vi "UA_Add node.vi"(8 "error in (no error)":errorcluster caption="错误输入（无错误）", 9 "XML Folder":T2[](array[typedef]), 11 "OPC UA server refnum in":refnum<k21>) -> (0 "error out":errorcluster caption="错误输出", 3 "OPC UA server refnum out":refnum<k21>)   [LabVIEW 2013, in "OPCUA XML.lvlib"]
uses:
  OPCUA XML.lvlib
  UA_XML Data.ctl
  UA_RowType.ctl
  UA_Node.ctl
  UA_OP Action.ctl
  <vilib>/OPCUA/NI OPC UA Server.lvlib
panel:
  out "node out":T1
  out "Data":string
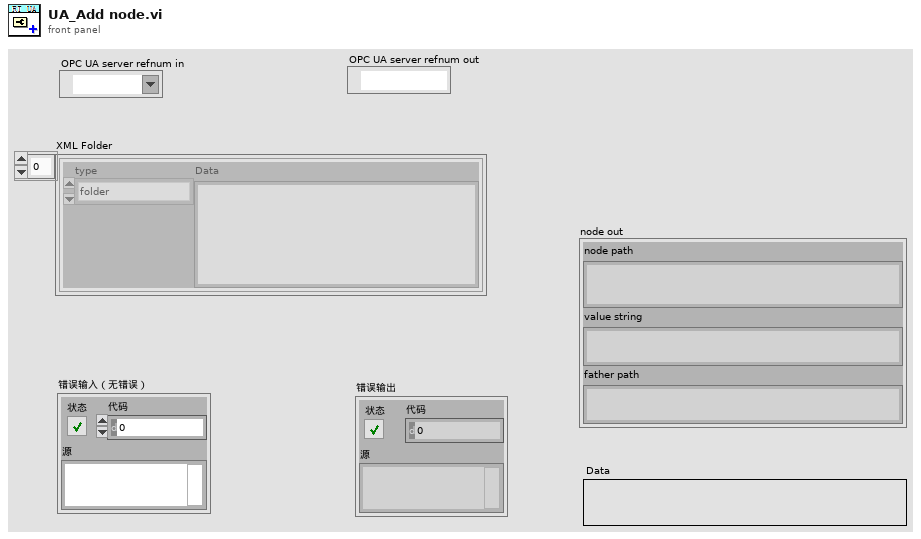
[diagram p1: front panel]
types:
  T1 = typedef "OPCUA XML.lvlib/UA_Node.ctl" = cluster{"node path":string, "value string":string, "father path":string}
  T2 = typedef "OPCUA XML.lvlib/UA_XML Data.ctl" = cluster{"type":T3, "Data":string}
  T3 = typedef "OPCUA XML.lvlib/UA_RowType.ctl" = enum16{"none", "folder", "item", "property", "folder end", "item end"}
  T4 = typedef "OPCUA XML.lvlib/UA_OP Action.ctl" = enum16{"Initial", "Add node", "Get node", "Get length", "View node"}
  T5 = cluster{"name":string, "data type":u16, "access level":u16, "description":string}
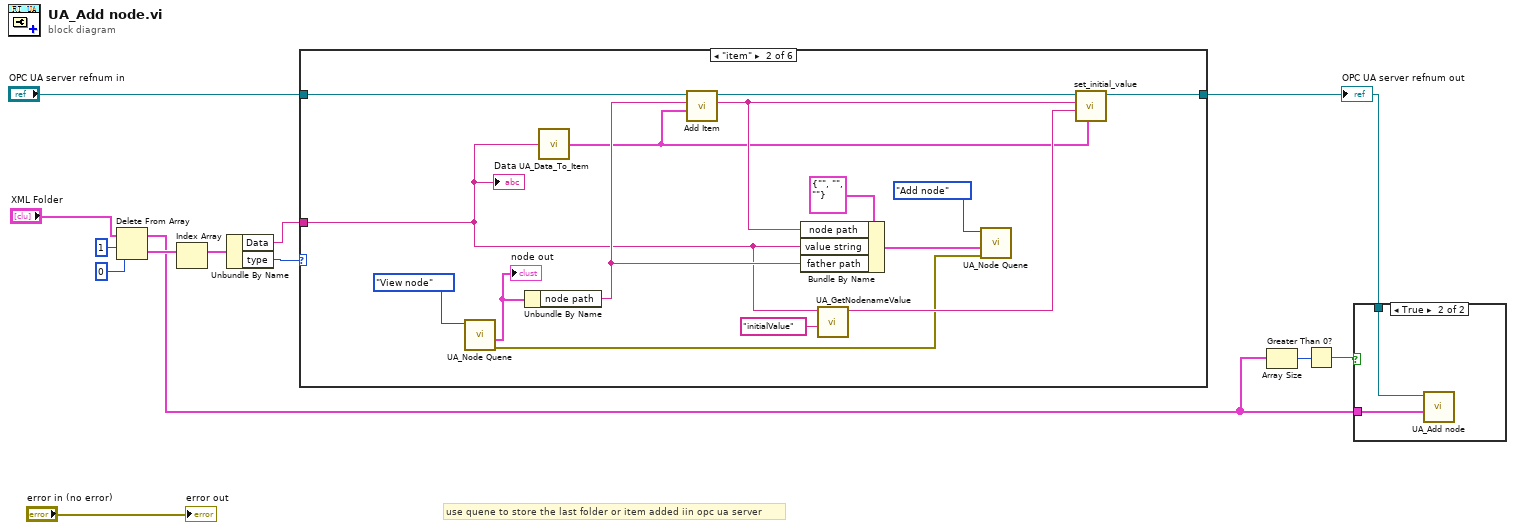
[diagram p0: block diagram]
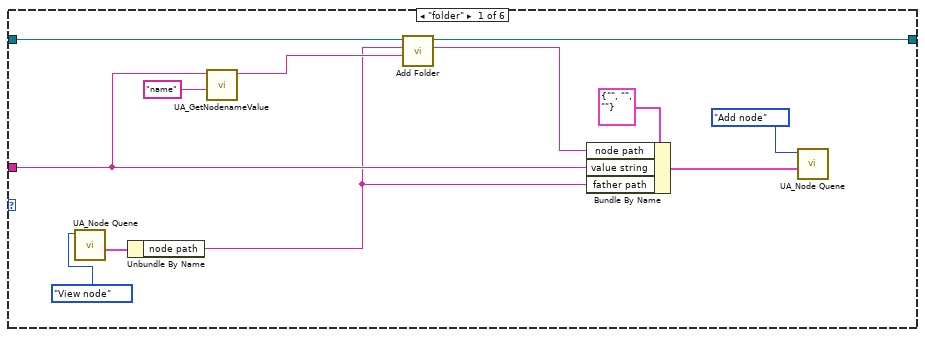
[diagram p3: hidden frame]
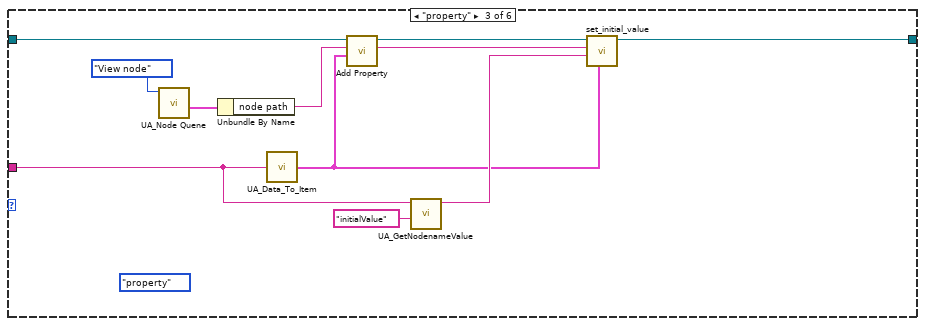
[diagram p4: hidden frame]
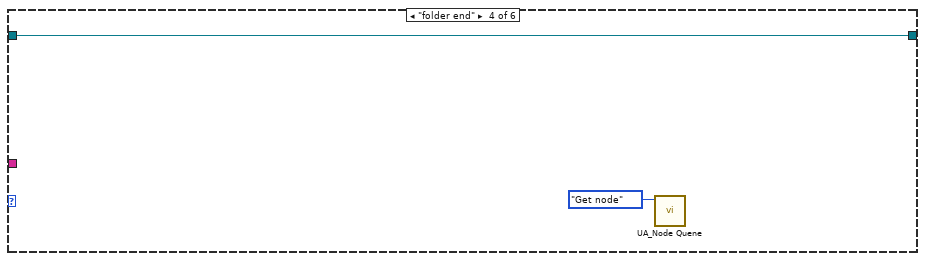
[diagram p5: hidden frame]
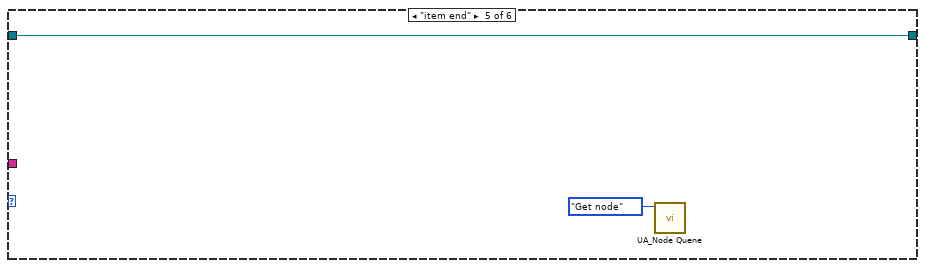
[diagram p6: hidden frame]
diagram:
  # "use quene to store the last folder or item added iin opc ua server"
  n1 = Delete From Array(array="XML Folder", length=1 ("长度"), index=0 ("索引")) -> (deleted portion=w10:T2[], array with subset deleted=w1:T2[])
  n2 = Index Array(array=w10) -> (element=w2:T2)  [unwired: 1 in]
  n3 = Unbundle By Name(w2) -> ("Data"=w7:string, "type"=w9:T3)
  n4 = case shown="\"item\"" w9 {
    tunnel: "OPC UA server refnum in" -> [w25 w40 w51 w53 w55 w56]
    tunnel: [w24 w31 w45 w53 w55 w56] -> w6
    tunnel: w7 -> [w16 w29 w44 _ _ _]
    frame "folder" {
      n5 = call "UA_Node Quene.vi"("OP Action"=UA_OP_Action."View node") -> ("node out"=w19:T1)  [unwired: 8 in, 2 out]
      n6 = Unbundle By Name(w19) -> ("node path"=w14:string)
      n7 = call "UA_GetNodenameValue.vi"("node name"="name", "Data"=w16) -> ("value"=w15:string)  [unwired: 9 in]
      n8 = call <vilib>:"Add Folder.vi"("folder name"=w15, "parent folder path"=w14, "OPC UA server refnum in"=w25) -> ("folder path"=w18:string, "OPC UA server refnum out"=w24:refnum<k21>)  [unwired: 5 in, 1 out]
      n9 = Bundle By Name(cluster=T1 {"node path"="", "value string"="", "father path"=""} ("Add node"), "node path"=w18, "value string"=w16, "father path"=w14) -> (w22:T1)
      n10 = call "UA_Node Quene.vi"("node in"=w22, "OP Action"=UA_OP_Action."Add node") -> ()  [unwired: 7 in, 3 out]
    }
    frame "item" {
      n11 = call "UA_Node Quene.vi"("OP Action"=UA_OP_Action."View node") -> ("error out"=w26:errorcluster, "node out"=w36:T1)  [unwired: 8 in, 1 out]
      "node out" <- w36
      n12 = Unbundle By Name(w36) -> ("node path"=w35:string)
      n13 = call "UA_Data_To_Item.vi"("data"=w29) -> ("item"=w27:T5)
      n14 = call <vilib>:"Add Item.vi"("item"=w27, "parent folder path"=w35, "OPC UA server refnum in"=w40) -> ("item path"=w32:string, "OPC UA server refnum out"=w33:refnum<k21>)  [unwired: 5 in, 1 out]
      n15 = Bundle By Name(cluster=T1 {"node path"="", "value string"="", "father path"=""} ("Add node"), "node path"=w32, "value string"=w29, "father path"=w35) -> (w38:T1)
      n16 = call "UA_GetNodenameValue.vi"("node name"="initialValue", "Data"=w29) -> ("value"=w28:string)  [unwired: 9 in]
      n17 = call "UA_Node Quene.vi"("error in (no error)"=w26, "node in"=w38, "OP Action"=UA_OP_Action."Add node") -> ()  [unwired: 6 in, 3 out]
      n18 = call "set_initial_value.vi"("item"=w27, "value string"=w28, "node path"=w32, "OPC UA server refnum in"=w33) -> ("OPC UA server refnum out"=w31:refnum<k21>)  [unwired: 5 in, 2 out]
      "Data" <- w29
    }
    frame "property" {
      (unwired) UA_RowType."property" ("data type")
      n19 = call "UA_Node Quene.vi"("OP Action"=UA_OP_Action."View node") -> ("node out"=w49:T1)  [unwired: 8 in, 2 out]
      n20 = Unbundle By Name(w49) -> ("node path"=w50:string)
      n21 = call "UA_Data_To_Item.vi"("data"=w44) -> ("item"=w41:T5)
      n22 = call <vilib>:"Add Property.vi"("property"=w41, "item path"=w50, "OPC UA server refnum in"=w51) -> ("property path"=w47:string, "OPC UA server refnum out"=w46:refnum<k21>)  [unwired: 5 in, 1 out]
      n23 = call "UA_GetNodenameValue.vi"("node name"="initialValue", "Data"=w44) -> ("value"=w42:string)  [unwired: 9 in]
      n24 = call "set_initial_value.vi"("item"=w41, "value string"=w42, "node path"=w47, "OPC UA server refnum in"=w46) -> ("OPC UA server refnum out"=w45:refnum<k21>)  [unwired: 5 in, 2 out]
    }
    frame "folder end" {
      n25 = call "UA_Node Quene.vi"("OP Action"=UA_OP_Action."Get node") -> ()  [unwired: 8 in, 3 out]
    }
    frame "item end" {
      n26 = call "UA_Node Quene.vi"("OP Action"=UA_OP_Action."Get node") -> ()  [unwired: 8 in, 3 out]
    }
    frame "none", Default {
    }
  }
  "OPC UA server refnum out" <- w6
  n27 = Array Size(array=w1) -> (size(s)=w5:i32)
  n28 = Greater Than 0?(x=w5) -> (x > 0?=w4:bool)
  n29 = case shown="True" w4 {
    tunnel: w6 -> [_ w58]
    tunnel: w1 -> [_ w57]
    frame False {
    }
    frame True {
      n30 = call "UA_Add node.vi"("XML Folder"=w57, "OPC UA server refnum in"=w58) -> ()  [unwired: 8 in, 2 out]
    }
  }
  "error out" <- "error in (no error)"
